vi "stop.vi"(8 "error in (no error)":errorcluster, 11 "WriteSignalsGenericPlugin in":refnum<class "SignalWriterDL101123SoundCard.lvclass">) -> (0 "error out":errorcluster, 3 "WriteSignalsGenericPlugin out":refnum<class "SignalWriterDL101123SoundCard.lvclass">)   [LabVIEW 2010, in "SignalWriterDL101123SoundCard.lvclass"]
uses:
  SignalWriterDL101123SoundCard.lvclass
  SignalWriterDL101123SoundCard.lvclass/SignalWriterDL101123SoundCard.ctl
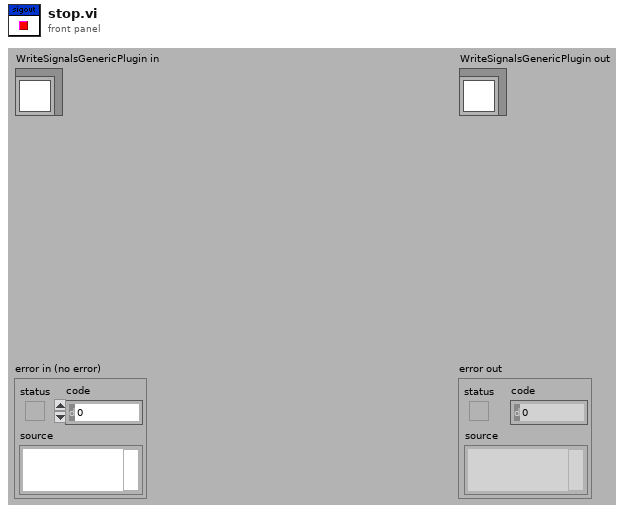
[diagram p1: front panel]
types:
  T1 = typedef "Sound Output Task ID.ctl" = u32
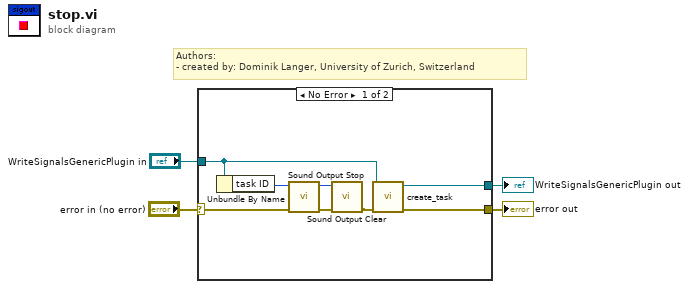
[diagram p0: block diagram]
diagram:
  # "Authors: \n- created by: Dominik Langer, University of Zurich, Switzerland"
  n1 = case shown="No Error" "error in (no error)" {
    selector: "error in (no error)" -> [w12 w14]
    tunnel: "WriteSignalsGenericPlugin in" -> [w6 w13]
    tunnel: [w10 w14] -> w2
    tunnel: [w5 w13] -> w1
    frame No Error {
      n2 = Unbundle By Name(w6) -> ("task ID"=w11:T1)
      n3 = call <vilib>:"Sound Output Stop.vi"("error in (no error)"=w12, "task ID"=w11) -> ("error out"=w9:errorcluster, "task ID out"=w7:T1)  [unwired: 8 in]
      n4 = call <vilib>:"Sound Output Clear.vi"("error in (no error)"=w9, "task ID"=w7) -> ("error out"=w8:errorcluster)  [unwired: 9 in]
      n5 = call-dynamic "create_task.vi"("error in (no error)"=w8, "SignalWriterDL101123SoundCard in"=w6) -> ("error out"=w10:errorcluster, "SignalWriterDL101123SoundCard out"=w5:refnum<class "SignalWriterDL101123SoundCard.lvclass">)  [unwired: 8 in]
    }
    frame Error {
    }
  }
  "error out" <- w2
  "WriteSignalsGenericPlugin out" <- w1
